vi "Build Command-Single Val.vi"(7 "error in":errorcluster, 8 "Val":string, 9 "Cmd":string, 10 "CN79000 in":refnum<class "CN79000.lvclass">) -> (0 "error out":errorcluster, 1 "DataOut":string[](array[string]), 2 "CommandStr":string[](array[string]), 3 "CN79000 out":refnum<class "CN79000.lvclass">)   [LabVIEW 2012, in "CN79000.lvclass"]
uses:
  CN79000.lvclass
  CN79000.lvclass/CN79000.ctl
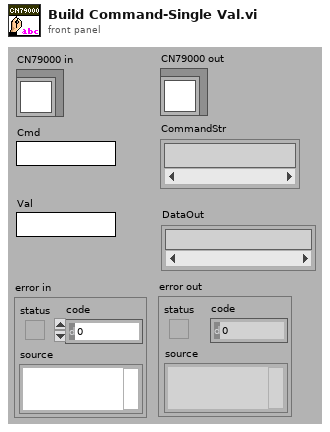
[diagram p1: front panel]
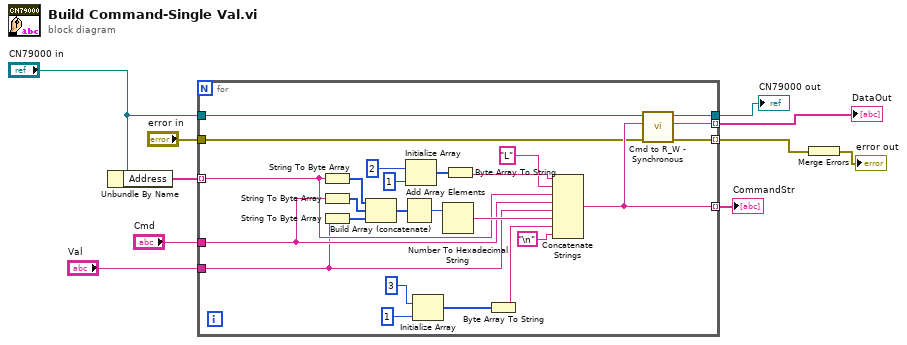
[diagram p0: block diagram]
diagram:
  n1 = Unbundle By Name("CN79000 in") -> ("Address"=w10:string[])
  n2 = for {
    tunnel: [w16] -> w9 mode=indexing
    tunnel: w10 -> [w19] mode=indexing
    tunnel: "Cmd" -> [w18]
    tunnel: "Val" -> [w17]
    tunnel: "CN79000 in" -> [w15]
    tunnel: [w14] -> w6
    tunnel: [w13] -> w2 mode=indexing
    tunnel: "error in" -> [w12]
    tunnel: [w11] -> w4 mode=indexing
    n3 = String To Byte Array(string=w19) -> (unsigned byte array=w34:u8[])
    n4 = String To Byte Array(string=w18) -> (unsigned byte array=w33:u8[])
    n5 = String To Byte Array(string=w17) -> (unsigned byte array=w30:u8[])
    n6 = Build Array (concatenate)(w34, w33, w30) -> (w32:u8[])
    n7 = Add Array Elements(numeric array=w32) -> (sum=w31:u8)
    n8 = Initialize Array(u8 2, 1 ("dimension size")) -> (w25:u8[])
    n9 = Initialize Array(u8 3, 1 ("dimension size")) -> (w24:u8[])
    n10 = Number To Hexadecimal String(2:w31) -> (0:w35:string)  [unwired: 1 in]
    n11 = Byte Array To String(unsigned byte array=w25) -> (string=w21:string)
    n12 = Byte Array To String(unsigned byte array=w24) -> (string=w23:string)
    n13 = Concatenate Strings(w21, "L" ("string"), w19, w18, w17, w35, w23, "\n") -> (w16:string)
    n14 = call-dynamic "Cmd to R_W - Synchronous.vi"("error in"=w12, "write buffer"=w16, "Serial IO in"=w15) -> ("error out"=w11:errorcluster, "read buffer"=w13:string, "Serial IO out"=w14:refnum<class "CN79000.lvclass">)  [unwired: 6 in]
  }
  "CN79000 out" <- w6
  "CommandStr" <- w9
  "DataOut" <- w2
  n15 = Merge Errors(w4) -> (→"error out":errorcluster)
